vi "Read File from Server.vi"(8 "error in (no error)":errorcluster, 9 "FileSize":i64, 10 "Local FilePath":path, 11 "FTP in":refnum<class "FTP.lvclass">) -> (0 "error out":errorcluster, 3 "FTP out":refnum<class "FTP.lvclass">)   [LabVIEW 2014, in "FTP.lvlib" / "FTP.lvclass"]
uses:
  FTP.lvclass
  controls/File Transfer Status.ctl
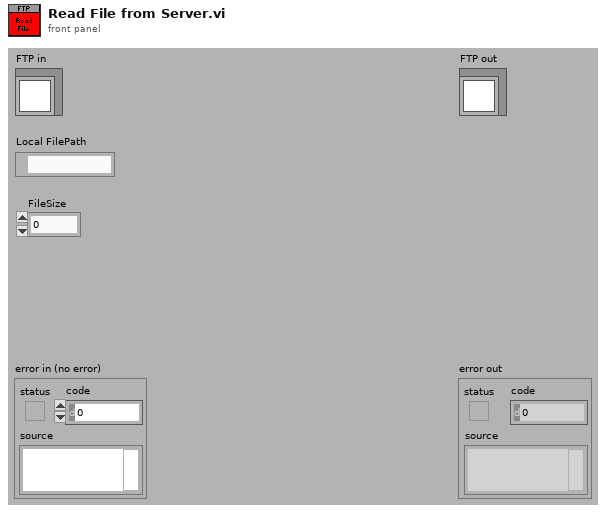
[diagram p1: front panel]
types:
  T1 = enum16{"open", "replace", "create", "open or create", "replace or create", "replace or create with confirmation"}
  T2 = typedef "FTP.lvlib/FTP.lvclass/File Transfer Status.ctl" = cluster{"File Name":string, "Percent Complete":u8, "File Size (in bytes)":i64, "Bytes Sent or Rcvd":i64}
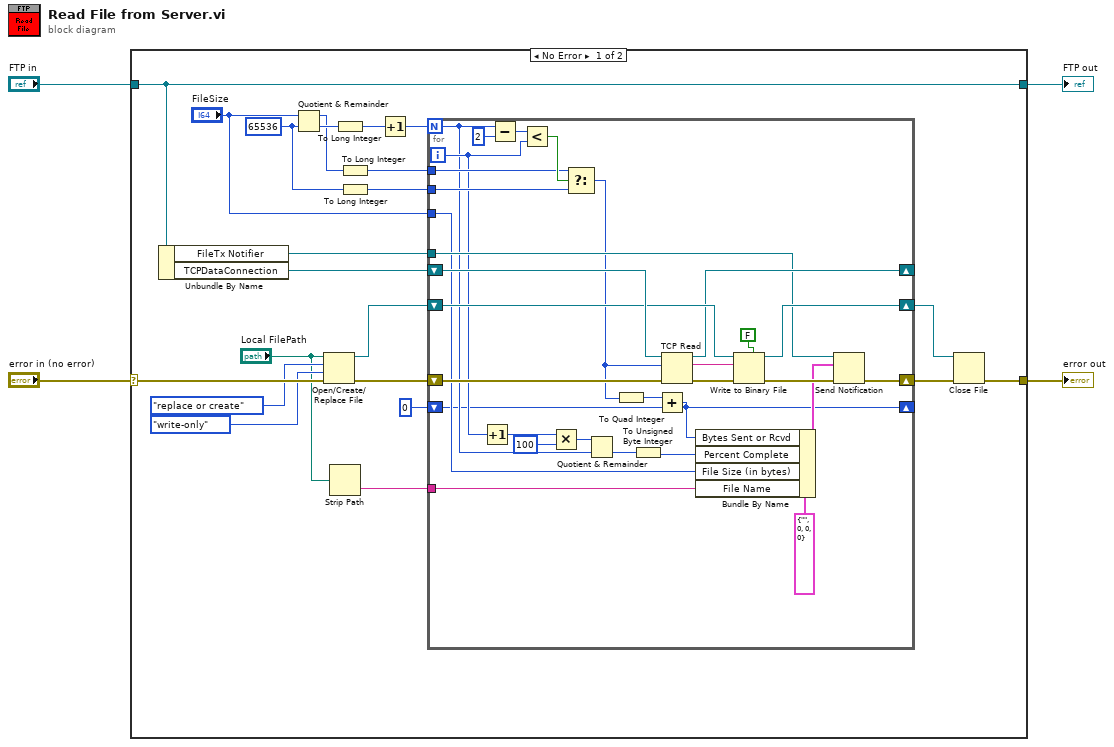
[diagram p0: block diagram]
diagram:
  n1 = case shown="No Error" "error in (no error)" {
    selector: "error in (no error)" -> [w26 w59]
    tunnel: [w18 w59] -> w3
    tunnel: [w24 w58] -> w1
    tunnel: "FTP in" -> [w24 w58]
    frame No Error {
      w16 = i64 65536 ("y")
      n2 = Unbundle By Name(w24) -> ("FileTx Notifier"=w9:refnum<notifier>, "TCPDataConnection"=w23:refnum<k5>)
      n3 = Quotient & Remainder(x="FileSize", y=w16) -> (x-y*floor(x/y)=w14:i64, floor(x/y)=w17:i64)
      n4 = Open/Create/Replace File(file path (use dialog)="Local FilePath", error in=w26, operation (0:open)=T1."replace or create", access (0:read/write)=enum16{"read/write", "read-only", "write-only"}."write-only") -> (refnum out=w21:refnum<file>, error out=w22:errorcluster)  [unwired: 2 in, 1 out]
      n5 = Strip Path(path="Local FilePath") -> (name=w7:string)  [unwired: 1 out]
      n6 = To Long Integer(number=w17) -> (32bit integer=w15:i32)
      n7 = To Long Integer(number=w14) -> (32bit integer=w12:i32)
      n8 = To Long Integer(number=w16) -> (32bit integer=w11:i32)
      n9 = Increment(x=w15) -> (x+1=w13:i32)
      n10 = for {
        N: w13 -> [w33]
        shift-right: [w51] -> w19
        shift-left: w21 -> [w54]
        shift-right: [w53] -> _
        shift-left: w23 -> [w56]
        shift-right: [w38] -> w20
        shift-left: w22 -> [w57]
        tunnel: w12 -> [w47]
        tunnel: w11 -> [w46]
        tunnel: w9 -> [w36]
        tunnel: w7 -> [w35]
        tunnel: "FileSize" -> [w31]
        shift-right: [w29] -> _
        shift-left: i64 0 -> [w30]
        i -> [w34]
        n11 = Increment(x=w34) -> (x+1=w43:i32)
        n12 = Subtract(x=w33, y=2) -> (x-y=w49:i32)
        n13 = Less?(x=w49, y=w34) -> (x < y?=w48:bool)
        n14 = Multiply(x=w43, y=100) -> (x*y=w42:i32)
        n15 = Select(t=w47, s=w48, f=w46) -> (s? t:f=w28:i32)
        n16 = Quotient & Remainder(x=w42, y=w33) -> (floor(x/y)=w41:i32)  [unwired: 1 out]
        n17 = To Quad Integer(1:w28) -> (0:w27:i64)
        n18 = To Unsigned Byte Integer(number=w41) -> (unsigned 8bit integer=w40:u8)
        n19 = Add(x=w27, y=w30) -> (x+y=w29:i64)
        n20 = TCP Read(connection ID=w56, bytes to read=w28, error in (no error)=w57) -> (connection ID out=w53:refnum<k5>, data out=w52:string, error out=w55:errorcluster)  [unwired: 2 in]
        n21 = Bundle By Name(cluster=T2 {"File Name"="", "Percent Complete"=0, "File Size (in bytes)"=0, "Bytes Sent or Rcvd"=0} ("notification"), "Bytes Sent or Rcvd"=w29, "Percent Complete"=w40, "File Size (in bytes)"=w31, "File Name"=w35) -> (w37:T2)
        n22 = Write to Binary File(file (use dialog)=w54, data=w52, error in=w55, 5:FALSE ("prepend array or string size? (T)")) -> (refnum out=w51:refnum<file>, error out=w39:errorcluster)  [unwired: 2 in, 1 out]
        n23 = Send Notification(notification=w37, notifier=w36, error in (no error)=w39) -> (error out=w38:errorcluster)  [unwired: 1 out]
      }
      n24 = Close File(refnum=w19, error in=w20) -> (error out=w18:errorcluster)  [unwired: 1 out]
    }
    frame Error {
    }
  }
  "error out" <- w3
  "FTP out" <- w1
